vi "Dashboard Main.vi"() -> ()   [LabVIEW 2012]
uses:
  <vilib>/event_ctls.llb/eventvkey.ctl
  <vilib>/Utility/config.llb/Read Key (String).vi
  <vilib>/Utility/config.llb/Read Key (I32).vi
  <vilib>/Utility/config.llb/Write Key (String).vi
  <vilib>/Utility/config.llb/Write Key (I32).vi
  <vilib>/Utility/config.llb/NI_LVConfig.lvlib
panel:
  out "Battery Value":dbl(slide) scale=0.0..14.0 scale format="%#_2e"
  out "Battery":sgl(graph)
  in  "Camera Settings":T1={"Frate Rate"=30, "Compression"=30, "Size"=1} {"Frate Rate" scale=1.0..30.0; "Size" items=["640x480", "320x240", "160x120"]}
  out "Mode":T2(ring)=enum."Auto Disabled"
  out "Camera IP":string
  out "JS1 Z":dbl(slide) scale=-1.0..1.0 scale format="%#_2e"
  out "JS2 Z":dbl(slide) scale=-1.0..1.0 scale format="%#_2e"
  out "Joystick 1":cluster{"X":dbl, "Y":dbl}[](graph)
  out "Joystick 2":cluster{"X":dbl, "Y":dbl}[](graph)
  out "JS Buttons 1":T3
  out "JS Buttons 2":T3
  out "MotorSlide4":dbl(slide) scale=-1.0..1.0 scale format="%#_2e"
  out "MotorSlide3":dbl(slide) scale=-1.0..1.0 scale format="%#_2e"
  out "MotorSlide2":dbl(slide) scale=-1.0..1.0 scale format="%#_2e"
  in  "MotorName3":string="Front Left"
  in  "MotorName4":string="Front Right"
  in  "MotorName1":string="Rear Left"
  in  "MotorName2":string="Rear Right"
  out "MotorChart4":dbl(graph)
  out "MotorChart3":dbl(graph)
  out "MotorChart2":dbl(graph)
  out "MotorSlide1":dbl(slide) scale=-1.0..1.0 scale format="%#_2e"
  out "MotorChart1":dbl(graph)
  out "Robot IP":string
  in  "Dashboard Tab":T4(tab)
  in  "Checkbox 2":bool
  in  "Checkbox 1":bool
  in  "Slider 1":dbl(slide) scale=0.0..100.0
  in  "Target Choice":i8(knob) scale=0.0..2.0
  out "Numeric Target Info":dbl[](array[numeric])
  out "Image Out":T5(plugin-control)
  in  "Slider":dbl(slide) scale=0.0..100.0 scale format="%#_3g"
  in  "On/Off":bool caption="Solenoid"
  in  "Test Name":u16(ring) items=["Select the test to run...", "Example Test", "-------------------------------", "List of tests is built in robot code.", "Replace with your own automated tests."]
  in  "Test Tree":string(tree)
  in  "Motor":cluster{"Value":dbl, "Enable":bool} {"Value" scale=-1.0..1.0 scale format="%#_3g"}
  out "Progress":T6 {"Test Progress" scale=0.0..100.0}
  in  "Rev/Fwd":cluster{"Forward":bool, "Reverse":bool}
  in  "Ring":u16(ring) items=["Auto", "Fixed indoor", "Fixed outdoor 1", "Fixed outdoor 2", "Fixed fluorescent 1", "Fixed fluorescent 2", "Hold current"]
  in  "Listbox":i32(listbox)
  in  "Viewer":T7(tab)
  out "Mbps":dbl format="%#.1g"
  in  "Enable":bool
  in  "DB Camera Config":bool
  out "Mbps":bool
  out "fps":dbl format="%#.1g"
  out "Image Error Message":string="Timeout in Camera Communications"
  out "Camera Image":T5(plugin-control)
  out "Center Target":bool
  out "Buttons 1":cluster{"1":bool, "2":bool, "3":bool}
  out "Kinect 1":cluster{"X":dbl, "Y":dbl, "Z":dbl} {"X" scale=1.0..-1.0; "Y" scale=1.0..-1.0; "Z" scale=1.0..-1.0}
  out "Buttons 2":cluster{"1":bool, "2":bool, "3":bool}
  out "Kinect 2":cluster{"X":dbl, "Y":dbl, "Z":dbl} {"X" scale=1.0..-1.0; "Y" scale=1.0..-1.0; "Z" scale=1.0..-1.0}
  out "Version":string
  out "Skeleton Picture":picture
  out "Players":i8
  out "Tree":string(tree)
  # "Drive & Motors"
  # "Robot IP:"
  # "Customize by placing controls and indicators here and name to match\nDashboard Variables on robot."
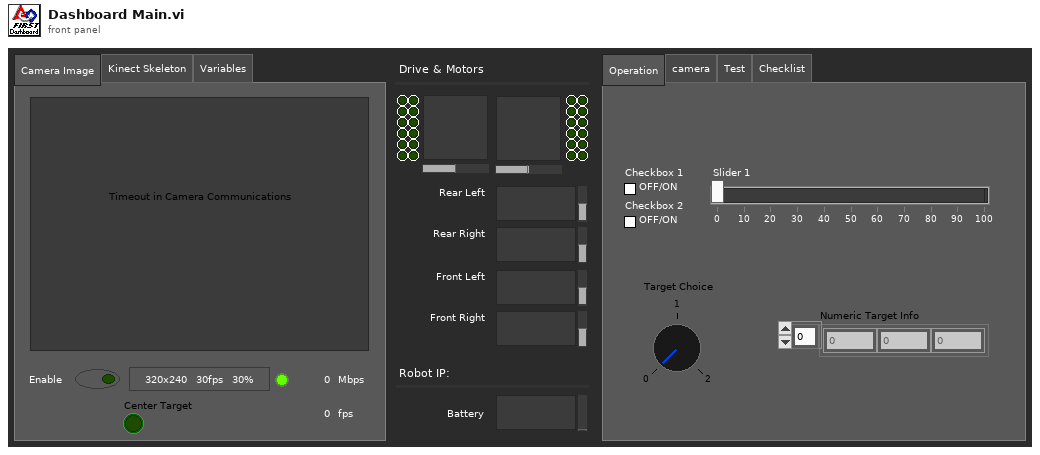
[diagram p1: front panel]
types:
  T1 = cluster{"Frate Rate":i32, "Compression":i32, "Size":u16}
  T2 = enum8{"Tele-Op Disabled", "Tele-Op Enabled", "Auto Disabled", "Auto Enabled", "Test Disabled", "Test Enabled", ""}
  T3 = cluster{bool, bool, bool, bool, bool, bool, bool, bool, bool, bool, bool, bool}
  T4 = enum32{"Operation", "camera", "Test", "Checklist"}
  T5 = typedef "IMAQ Image.ctl" = refnum<image>
  T6 = cluster{"Test Progress":u8, "Test Progress Text":string}
  T7 = enum32{"Camera Image", "Kinect Skeleton", "Variables"}
  T8 = typedef "Image Type" = u32
  T9 = typedef "LVBoundsTypeDef.ctl" = cluster{"Width":u32, "Height":u32}
  T10 = typedef "SkeletonTrackState.ctl" = enum32{"NotTracked", "PositionOnly", "Tracked"}
  T11 = cluster{"TrackingState":u8[], "Position":cluster{"x":sgl, "y":sgl, "z":sgl}, cluster{"x":sgl, "y":sgl, "z":sgl, sgl}[], "TrackState":T10}
  T12 = cluster{cluster{"ScaledToPercentRange":dbl, "ScaledToPercentRange":dbl, "ScaledToPercentRange":dbl}, cluster{bool, bool, bool}}[]
  T13 = cluster{cluster{"ScaledToPercentRange":dbl, "ScaledToPercentRange":dbl, "ScaledToPercentRange":dbl}, cluster{bool, bool, bool}}
  T14 = cluster{"ScaledToPercentRange":dbl, "ScaledToPercentRange":dbl, "ScaledToPercentRange":dbl}
  T15 = typedef "LVRectTypeDef.ctl" = cluster{"Left":i16, "Top":i16, "Right":i16, "Bottom":i16}
  T16 = cluster{"Competition mode":bool, "Robot Link":bool, "Autonomous":bool, "Enabled":bool, "E-Stop":bool, "Simulated":bool, "TestMode":bool, "Docked Window":bool}
  T17 = cluster{"Boolean Array[0]":bool, "Boolean Array[1]":bool, "Boolean Array[2]":bool, "Boolean Array[3]":bool, "Boolean Array[4]":bool, "Boolean Array[5]":bool, "Boolean Array[6]":bool, "Boolean Array[7]":bool, "Boolean Array[8]":bool, "Boolean Array[9]":bool, "Boolean Array[10]":bool, "Boolean Array[11]":bool}
  T18 = typedef "NI_LVConfig.lvlib/Config Data RefNum.ctl" = refnum<k1>
  T19 = typedef "eventvkey.ctl" = enum16{"ASCII", "Enter", "Return", "Shift", "Ctrl", "Alt", "Cmd", "Opt", "Caps", "NumLock", "Clear", "Break", "Up", "Down", "Left", "Right", "Insert", "Delete", "Home", "End", "PageUp", "PageDown", "Escape", "Help", "Pause", "ScrollLock", "F1", "F2", "F3", "F4", "F5", "F6", "F7", "F8", "F9", "F10", "F11", "F12", "F13", "F14", "F15", "F16", "F17", "F18", "F19", "F20", "F21", "F22", "F23", "F24", "Play", "VolumeUp", "VolumeDown", "Mute", "Two Byte Char"}
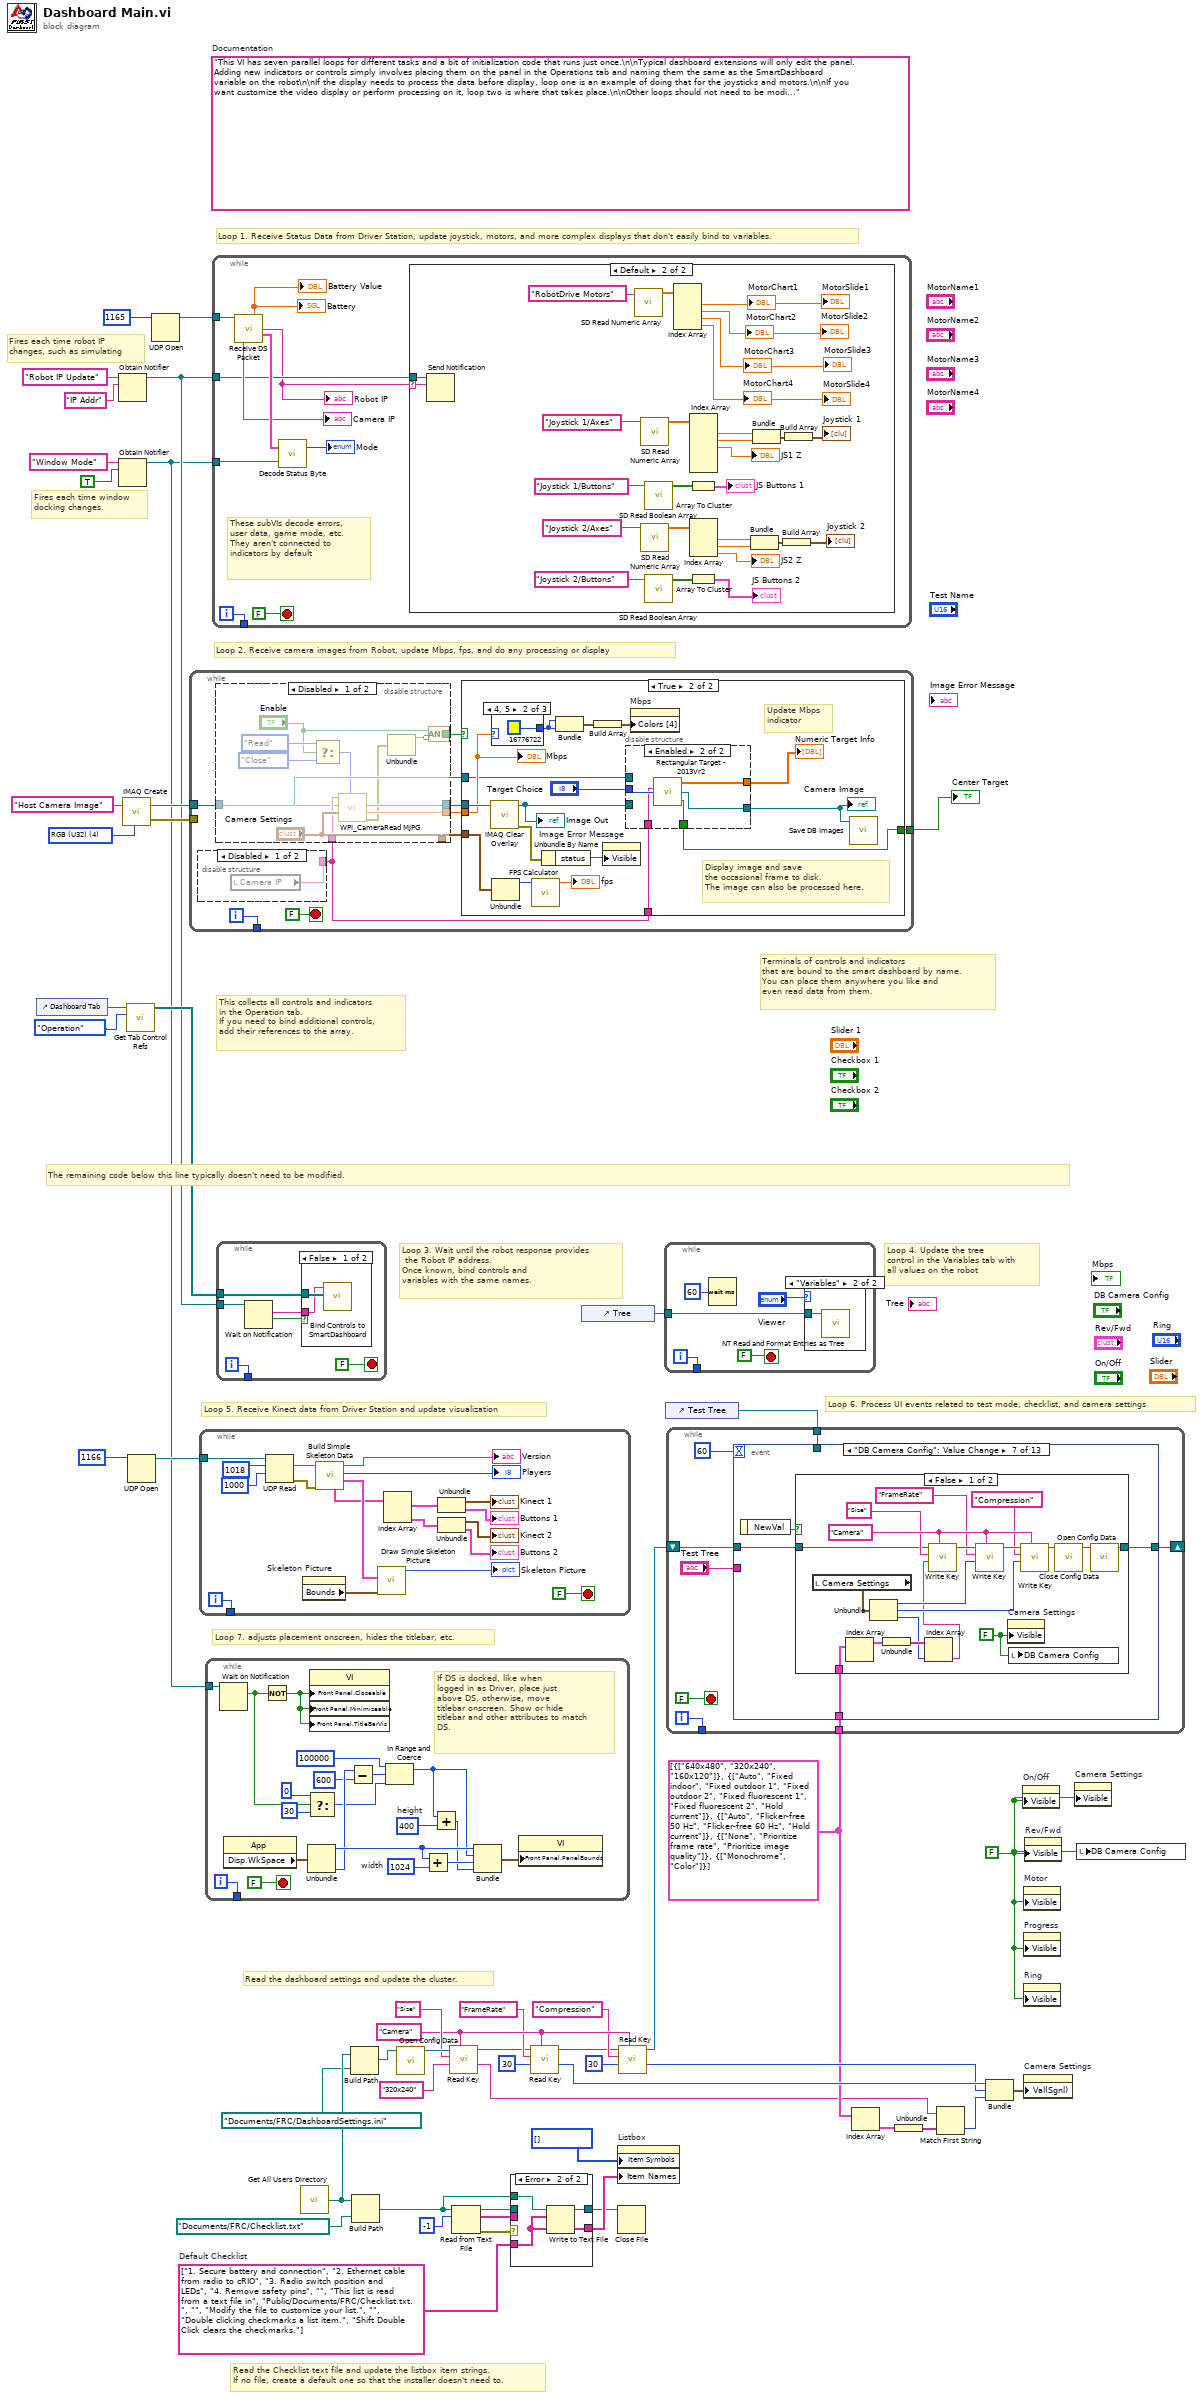
[diagram p0: block diagram]
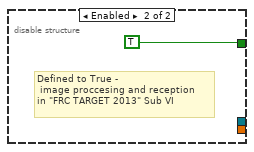
[diagram p3: hidden frame]
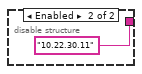
[diagram p4: hidden frame]
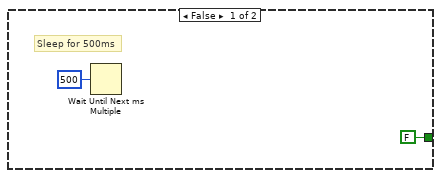
[diagram p5: hidden frame]
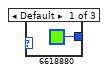
[diagram p7: hidden frame]
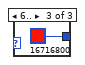
[diagram p8: hidden frame]
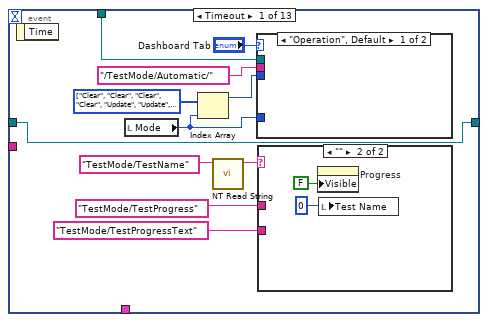
[diagram p10: hidden frame]
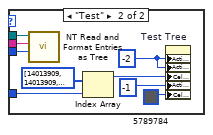
[diagram p11: hidden frame]
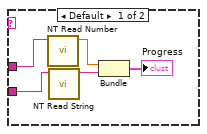
[diagram p12: hidden frame]
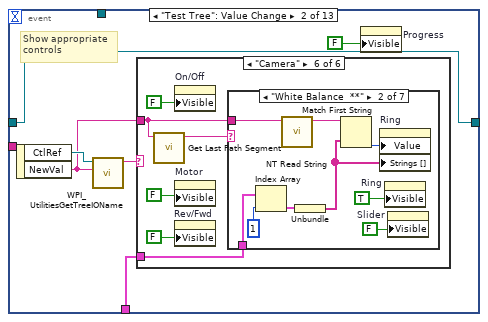
[diagram p13: hidden frame]
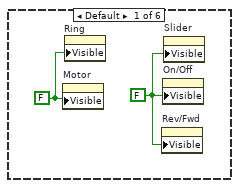
[diagram p14: hidden frame]
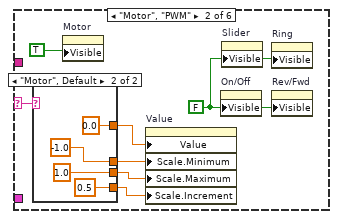
[diagram p15: hidden frame]
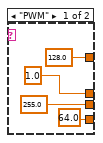
[diagram p16: hidden frame]
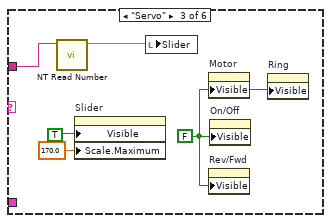
[diagram p17: hidden frame]
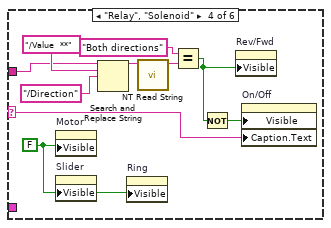
[diagram p18: hidden frame]
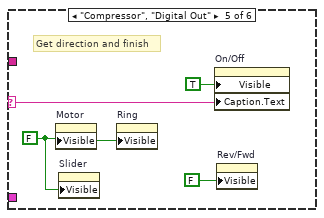
[diagram p19: hidden frame]
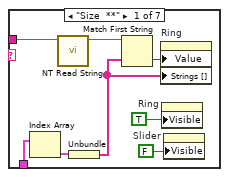
[diagram p20: hidden frame]
diagram:
  w22 = "Camera"
  w14 = cluster{string[]}[] [{["640x480", "320x240", "160x120"]}, {["Auto", "Fixed indoor", "Fixed outdoor 1", "Fixed outdoor 2", "Fixed fluorescent 1", "Fixed fluorescent 2", "Hold current"]}, {["Auto", "Flicker-free 50 Hz", "Flicker-free 60 Hz", "Hold current"]}, {["None", "Prioritize frame rate", "Prioritize image quality"]}, {["Monochrome", "Color"]}]
  w30 = string[] ["1. Secure battery and connection", "2. Ethernet cable from radio to cRIO", "3. Radio switch position and LEDs", "4. Remove safety pins", "", "This list is read from a text file in", "Public/Documents/FRC/Checklist.txt.", "", "Modify the file to customize your list.", "", "Double clicking checkmarks a list item.", "Shift Double Click clears the checkmarks."]  # Default Checklist
  w28 = FALSE ("Visible")
  (unwired) "This VI has seven parallel loops for different tasks and a bit of initialization code that runs just once.\n\nTypical dashboard extensions will only edit the panel. Adding new indicators or controls simply involves placing them on the panel in the Operations tab and naming them the same as the SmartDashboard variable on the robot\n\nIf the display needs to process the data before display, loop one is an example of doing that for the joysticks and motors.\n\nIf you want customize the video display or perform processing on it, loop two is where that takes place.\n\nOther loops should not need to be modified. They are pretty standard, and document the task they perform."  # Documentation
  w51 = T8 4 items=["Grayscale (U8)", "Grayscale (I16)", "Grayscale (SGL)", "Complex (CSG)", "RGB (U32)", "HSL (U32)", "RGB (U64)"] ("Image Type")
  # "Fires each time robot IP\nchanges, such as simulating"
  # "Fires each time window\ndocking changes."
  # "Read the Checklist text file and update the listbox item strings.\nIf no file, create a default one so that the installer doesn't need to."
  # "This collects all controls and indicators\nin the Operation tab.\nIf you need to bind additional controls,\nadd their references to the array."
  # "The remaining code below this line typically doesn't need to be modified."
  # "Loop 6. Process UI events related to test mode, checklist, and camera settings"
  # "Read the dashboard settings and update the cluster."
  # "Terminals of controls and indicators\nthat are bound to the smart dashboard by name.\nYou can place them anywhere you like and\neven read data from them."
  # "Loop 4. Update the tree\ncontrol in the Variables tab with\nall values on the robot"
  # "Loop 3. Wait until the robot response provides\n the Robot IP address.\nOnce known, bind controls and\nvariables with the same names."
  # "Loop 5. Receive Kinect data from Driver Station and update visualization"
  # "Loop 7. adjusts placement onscreen, hides the titlebar, etc."
  # "Loop 1. Receive Status Data from Driver Station, update joystick, motors, and more complex displays that don't easily bind to variables."
  # "Loop 2. Receive camera images from Robot, update Mbps, fps, and do any processing or display"
  n1 = control-ref of="Dashboard Tab"() -> (w44:refnum<vi>)
  n2 = Obtain Notifier(name (unnamed)="Robot IP Update", notification data type="IP Addr" ("name (unnamed)")) -> (notifier out=w41:refnum<notifier>)  [unwired: 2 in, 2 out]
  n3 = Obtain Notifier(name (unnamed)="Window Mode", notification data type=TRUE) -> (notifier out=w34:refnum<notifier>)  [unwired: 2 in, 2 out]
  n4 = call "IMAQ Create"("Image Name"="Host Camera Image", "Image Type"=w51) -> ("New Image"=w49:T5, "error out"=w48:errorcluster)  [unwired: 2 in, 1 out]
  n5 = call <vilib>:"Get Tab Control Refs.vi"("Page Index"=enum32{"Operation", "Test"}."Operation" ("Dashboard Tab"), "TabControl in"=w44) -> ("ControlsOnPage"=w45:refnum<vi>[])  [unwired: 9 in]
  n6 = UDP Open(11:u16 1166 ("port")) -> (port=w46:refnum<k16>)  [unwired: 2 in, 4 out]
  n7 = UDP Open(11:u16 1165 ("port")) -> (port=w52:refnum<k16>)  [unwired: 2 in, 4 out]
  n8 = while {
    tunnel: w49 -> [w56]
    tunnel: w48 -> [_]
    tunnel: [w61] -> _
    tunnel: [w54] -> w1
    i -> [w61]
    stop <- FALSE stop-if-true
    n9 = disable-structure shown="Disabled" {
      disable-tunnel: [w76 "10.22.30.11" ("camera IP")] -> w57
      frame Disabled {
        n10 = local read "Camera IP"() -> (w76:string)
      }
      frame Enabled {
      }
    }
    n11 = disable-structure shown="Disabled" {
      disable-tunnel: ["Camera Settings" _] -> w60
      disable-tunnel: [w73 _] -> w59
      disable-tunnel: [w72 _] -> w58
      disable-tunnel: [w65 TRUE] -> w55
      disable-tunnel: w57 -> [w64 _]
      disable-tunnel: w56 -> [w63 _]
      frame Disabled {
        n12 = Select(t=enum16{"Read", "Reopen", "Close"}."Read" ("Operation"), s="Enable", f=enum16{"Read", "Reopen", "Close"}."Close" ("Operation")) -> (s? t:f=w69:enum16{"Read", "Reopen", "Close"})
        n13 = call <vilib>:"WPI_CameraRead MJPG.vi"("Operation"=w69, "Camera Settings"="Camera Settings", "Image"=w63, "address"=w64) -> ("error out"=w68:errorcluster, "Bandwidth (kbps)"=w72:dbl, "Image Out"=w73:T5)  [unwired: 5 in]
        n14 = Unbundle(w68) -> ("status"=w66:bool)  [unwired: 2 out]
        n15 = Compound Arithmetic op=AND("Enable", invert w66) -> (w65:bool)
      }
      frame Enabled {
        # "Defined to True -\n image proccesing and reception \nin \"FRC TARGET 2013\" Sub VI"
      }
    }
    n16 = case shown="True" w55 {
      tunnel: w60 -> [_ w88]
      tunnel: w59 -> [_ w91]
      tunnel: w58 -> [_ w90]
      tunnel: w57 -> [_ w82]
      tunnel: w56 -> [_ w81]
      tunnel: [FALSE ("Center Target") w80] -> w54
      frame False {
        # "Sleep for 500ms"
        n17 = Wait Until Next ms Multiple(millisecond multiple=u32 500) -> ()  [unwired: 1 out]
      }
      frame True {
        # "Display image and save\nthe occasional frame to disk.\nThe image can also be processed here."
        # "Update Mbps\nindicator"
        n18 = call "IMAQ Clear Overlay"("Image"=w91) -> ("error out"=w95:errorcluster, "Image Out"=w85:T5)  [unwired: 2 in, 7 out]
        "Image Out" <- w85
        n19 = case shown="4, 5" w90 {
          tunnel: [u32 6618880 ("Color Box") u32 16776722 ("Color Box") u32 16716800 ("Color Box")] -> w92
          frame Default {
          }
          frame 4, 5 {
          }
          frame 6.. {
          }
        }
        n20 = Unbundle(w88) -> ("Frate Rate"=w87:i32)  [unwired: 2 out]
        n21 = call "FPS Calculator.vi"("Average Count"=w87) -> ("fps"=→"fps":dbl)  [unwired: 10 in]
        n22 = Unbundle By Name(w95) -> ("status"=w96:bool)
        n23 = Bundle("Color Box"=w92, "Color Box"=w92) -> (w94:cluster{"Color Box":u32, "Color Box":u32})  [unwired: 1 out]
        n24 = Build Array(w94) -> (w93:cluster{"Color Box":u32, "Color Box":u32}[])
        n25 = property on="Image Error Message" class="Str"("Visible"=w96) -> ()  [unwired: 2 in, 2 out]
        n26 = disable-structure shown="Enabled" {
          disable-tunnel: [w97 w102] -> w86
          disable-tunnel: w85 -> [w97 _]
          disable-tunnel: "Target Choice" -> [_ w101]
          disable-tunnel: [_ w100] -> w83
          disable-tunnel: w82 -> [_ w98]
          disable-tunnel: w81 -> [_ _]
          disable-tunnel: [_ w99] -> w80
          frame Disabled {
          }
          frame Enabled {
            n27 = call "Rectangular Target - 2013Vr2.vi"("Target Choice"=w101, "Camera IP Address"=w98) -> ("Center Target"=w99:bool, "Processed Image"=w102:T5, "Numeric Target Info"=w100:dbl[])  [unwired: 2 in]
          }
        }
        "Camera Image" <- w86
        "Numeric Target Info" <- w83
        n28 = property on="Mbps" class="Bool (strict)"("Colors [4]"=w93) -> ()  [unwired: 2 in, 2 out]
        n29 = call "Save DB Images.vi"("Image"=w86) -> ()  [unwired: 2 in, 1 out]
        "Mbps" <- w90
      }
    }
  }
  "Center Target" <- w1
  n30 = while {
    tunnel: w46 -> [w122]
    tunnel: [w107] -> _
    i -> [w107]
    stop <- FALSE stop-if-true
    n31 = UDP Read(connection ID=w122, max size (548)=1018 ("bytes to read"), timeout ms (25000)=1000) -> (data out=w116:string, error out=w106:errorcluster)  [unwired: 1 in, 3 out]
    n32 = property on="Skeleton Picture" class="Pict"() -> ("Bounds"=w118:T9)  [unwired: 2 in, 2 out]
    n33 = call "Build Simple Skeleton Data.vi"("error in (no error)"=w106, "data in"=w116) -> ("Skeleton Data"=w117:T11, "NumPlayers"=→"Players":i8, "Version String"=→"Version":string, "Simple Joystick Info"=w114:T12)  [unwired: 5 in, 1 out]
    n34 = call "Draw Simple Skeleton Picture.vi"("Bounds"=w118, "Simple Skeleton"=w117) -> ("new picture out"=→"Skeleton Picture":picture)  [unwired: 9 in]
    n35 = Index Array(array=w114) -> (element #1=w113:T13, element #2=w112:T13)  [unwired: 2 in]
    n36 = Unbundle(w113) -> (→"Kinect 1":T14, →"Buttons 1":cluster{bool, bool, bool})
    n37 = Unbundle(w112) -> (→"Kinect 2":T14, →"Buttons 2":cluster{bool, bool, bool})
  }
  n38 = while {
    tunnel: w34 -> [w143]
    tunnel: [w141] -> _
    i -> [w141]
    stop <- FALSE stop-if-true
    w133 = 1024  # width
    w136 = 400  # height
    # "If DS is docked, like when\nlogged in as Driver, place just\nabove DS, otherwise, move\ntitlebar onscreen. Show or hide\ntitlebar and other attributes to match\nDS."
    n39 = Wait on Notification(notifier=w143) -> (notification=w128:bool)  [unwired: 3 in, 3 out]
    n40 = property class="App"() -> ("Disp.WkSpace"=w139:T15)  [unwired: 2 in, 2 out]
    n41 = Not(x=w128) -> (.not. x?=w142:bool)
    n42 = Unbundle(w139) -> ("Left"=w137:i16, "Bottom"=w134:i16)  [unwired: 2 out]
    n43 = Select(t=0, s=w128, f=30) -> (s? t:f=w127:i32)
    n44 = property class="VI"("Front Panel.Closeable"=w142, "Front Panel.Minimizeable"=w142, "Front Panel.TitleBarVis"=w142) -> ()  [unwired: 2 in, 2 out]
    n45 = Subtract(x=w134, y=600) -> (x-y=w131:i32)
    n46 = In Range and Coerce(upper limit=100000, x=w131, lower limit=w127) -> (coerced(x)=w125:i32)  [unwired: 1 out]
    n47 = Add(x=w137, y=w133) -> (x+y=w138:i32)
    n48 = Add(x=w125, y=w136) -> (x+y=w135:i32)
    n49 = Bundle("Left"=w137, w125, w138, w135) -> (w140:cluster{"Left":i16, i32, i32, i32})  [unwired: 1 out]
    n50 = property class="VI"("Front Panel.PanelBounds"=w140) -> ()  [unwired: 2 in, 2 out]
  }
  n51 = while {
    tunnel: w52 -> [w152]
    tunnel: w41 -> [w146]
    tunnel: w34 -> [w150]
    tunnel: [w147] -> _
    i -> [w147]
    stop <- FALSE stop-if-true
    # "These subVIs decode errors, user data, game mode, etc.\nThey aren't connected to indicators by default"
    n52 = call "Receive DS Packet.vi"("Recv Socket"=w152) -> ("Battery"=→"Battery" →"Battery Value":sgl, "Robot IP Address"=w145:string, "Status"=w153:T16, "Camera IP Address"=→"Camera IP":string)  [unwired: 1 in, 10 out]
    "Robot IP" <- w145
    n53 = call "Decode Status Byte.vi"("Window Mode Notifier"=w150, "Status"=w153) -> ("Mode"=→"Mode":T2)  [unwired: 1 out]
    n54 = case shown="Default" w145 {
      selector: w145 -> [_ w155]
      tunnel: w146 -> [_ w156]
      frame "0.0.0.0" {
        # "Robot not responding, don't poll the variables"
      }
      frame Default {
        n55 = Send Notification(notification=w155, notifier=w156) -> ()  [unwired: 1 in, 2 out]
        n56 = call <vilib>:"SD Read Numeric Array.vi"("Name"="RobotDrive Motors") -> ("Numeric Array"=w179:dbl[])  [unwired: 8 in, 2 out]
        n57 = call <vilib>:"SD Read Numeric Array.vi"("Name"="Joystick 1/Axes") -> ("Numeric Array"=w172:dbl[])  [unwired: 8 in, 2 out]
        n58 = call <vilib>:"SD Read Numeric Array.vi"("Name"="Joystick 2/Axes") -> ("Numeric Array"=w166:dbl[])  [unwired: 8 in, 2 out]
        n59 = call <vilib>:"SD Read Boolean Array.vi"("Name"="Joystick 1/Buttons") -> ("Boolean Array"=w174:bool[])  [unwired: 8 in, 2 out]
        n60 = call <vilib>:"SD Read Boolean Array.vi"("Name"="Joystick 2/Buttons") -> ("Boolean Array"=w165:bool[])  [unwired: 8 in, 2 out]
        n61 = Index Array(array=w179) -> (element #1=→"MotorChart1" →"MotorSlide1":dbl, element #2=→"MotorSlide2" →"MotorChart2":dbl, element #3=→"MotorChart3" →"MotorSlide3":dbl, element #4=→"MotorChart4" →"MotorSlide4":dbl)  [unwired: 4 in]
        n62 = Array To Cluster(array=w174) -> (cluster=→"JS Buttons 1":T17)
        n63 = Array To Cluster(array=w165) -> (cluster=→"JS Buttons 2":T17)
        n64 = Index Array(array=w172) -> (element #1=w169:dbl, element #2=w170:dbl, element #3=→"JS1 Z":dbl)  [unwired: 6 in, 3 out]
        n65 = Index Array(array=w166) -> (element #1=w161:dbl, element #2=w160:dbl, element #3=→"JS2 Z":dbl)  [unwired: 3 in]
        n66 = Bundle("Numeric"=w161, "Numeric"=w160) -> (w162:cluster{"Numeric":dbl, "Numeric":dbl})  [unwired: 1 in]
        n67 = Bundle("Numeric"=w169, "Numeric"=w170) -> (w168:cluster{"Numeric":dbl, "Numeric":dbl})  [unwired: 1 in]
        n68 = Build Array(w162) -> (→"Joystick 2":cluster{"Numeric":dbl, "Numeric":dbl}[])
        n69 = Build Array(w168) -> (→"Joystick 1":cluster{"Numeric":dbl, "Numeric":dbl}[])
      }
    }
  }
  n70 = while {
    tunnel: w45 -> [w188]
    tunnel: w41 -> [w185]
    tunnel: [w183] -> _
    i -> [w183]
    stop <- FALSE stop-if-true
    n71 = Wait on Notification(notifier=w185) -> (notification=w184:string, timed out?=w186:bool)  [unwired: 3 in, 2 out]
    n72 = case shown="False" w186 {
      tunnel: w188 -> [w190 _]
      tunnel: w184 -> [w189 _]
      frame False {
        n73 = call <vilib>:"Bind Controls to SmartDashboard.vi"("Bound Control Refs"=w190, "Server IP Address"=w189) -> ()  [unwired: 10 in]
      }
      frame True {
      }
    }
  }
  n74 = call "Get All Users Directory.vi"() -> ("All User Path"=w27:path)
  n75 = Build Path(base path=w27, name or relative path=path "Documents/FRC/DashboardSettings.ini") -> (appended path=w26:path)
  n76 = Build Path(base path=w27, name or relative path=path "Documents/FRC/Checklist.txt") -> (appended path=w31:path)
  n77 = call <vilib>:"Open Config Data.vi"("configuration file path"=w26) -> ("refnum"=w25:T18)  [unwired: 8 in, 2 out]
  n78 = call-poly <vilib>:"Read Key.vi"("section"=w22, "default value"="320x240", "key"="Size", "refnum"=w25) -> ("value"=w12:string, "refnum out"=w7:T18)  [unwired: 2 in, 4 out]
  n79 = Read from Text File(file (use dialog)=w31, count=-1 ("timeout ms (25000)")) -> (refnum out=w9:refnum<file>, text=w32:string[], error out=w33:errorcluster)  [unwired: 2 in, 1 out]
  n80 = case shown="Error" w33 {
    tunnel: w32 -> [w192 _]
    tunnel: [w192 w194] -> w29
    tunnel: w30 -> [_ w194]
    tunnel: w31 -> [_ w195]
    tunnel: [w191 w193] -> w8
    tunnel: w9 -> [w191 _]
    frame No Error {
    }
    frame Error {
      n81 = Write to Text File(file (use dialog)=w195, text=w194) -> (refnum out=w193:refnum<file>)  [unwired: 2 in, 2 out]
    }
  }
  n82 = call-poly <vilib>:"Read Key.vi"("section"=w22, "default value"=30, "key"="FrameRate", "refnum"=w7) -> ("value"=w17:i32, "refnum out"=w6:T18)  [unwired: 1 in, 5 out]
  n83 = control-ref of="Tree"() -> (w3:refnum<vi>)
  n84 = property on="Listbox" class="LstBox (strict)"("Item Symbols"=i32[] [], "Item Names"=w29) -> ()  [unwired: 2 in, 2 out]
  n85 = Close File(refnum=w8) -> ()  [unwired: 1 in, 2 out]
  n86 = call-poly <vilib>:"Read Key.vi"("section"=w22, "default value"=30, "key"="Compression", "refnum"=w6) -> ("value"=w16:i32, "refnum out"=w4:T18)  [unwired: 1 in, 5 out]
  n87 = while {
    tunnel: [w197] -> _
    tunnel: w3 -> [w196]
    i -> [w197]
    stop <- FALSE stop-if-true
    n88 = Wait (ms)(milliseconds to wait=u32 60) -> ()  [unwired: 1 out]
    n89 = case shown="\"Variables\"" "Viewer" {
      tunnel: w196 -> [_ w201]
      frame Default {
      }
      frame "Variables" {
        n90 = call <vilib>:"NT Read and Format Entries as Tree.vi"("Tree Refnum"=w201) -> ()  [unwired: 9 in, 2 out]
      }
    }
  }
  n91 = control-ref of="Test Tree"() -> (w2:refnum<vi>)
  n92 = while {
    tunnel: w14 -> [w206]
    shift-right: [w205] -> _
    shift-left: w4 -> [w204]
    tunnel: [w203] -> _
    tunnel: w2 -> [w202]
    i -> [w203]
    stop <- FALSE stop-if-true
    n93 = event shown="[6] \"DB Camera Config\": Value Change" {
      selector: _ -> [_ _ _ _ _ _ _ _ _ _ _ _ _]
      dyn-events: _ -> [_ _ _ _ _ _ _ _ _ _ _ _ _]
      timeout: u32 60 ("milliseconds to wait") -> [_ _ _ _ _ _ _ _ _ _ _ _ _]
      tunnel: w202 -> [w216 _ _ _ _ _ _ _ _ _ _ _ _]
      tunnel: "Test Tree" -> [_ _ _ _ _ _ _ _ w410 w418 w420 w424 w432]
      tunnel: w206 -> [_ w238 _ _ _ _ w374 w404 _ _ _ _ _]
      tunnel: [w210 w237 _ w340 w348 w360 w373 w397 w409 w416 w419 w423 w431] -> w205
      tunnel: w204 -> [w210 w237 _ w340 w348 w360 w372 w397 w409 w416 w419 w423 w431]
      event Timeout {
        w215 = enum16{"Update", "Clear"}[] [enum."Clear", enum."Clear", enum."Clear", enum."Clear", enum."Update", enum."Update", enum."Clear"] items=["Update", "Clear"]
        n94 = event-data() -> ()  [unwired: 1 in, 1 out]
        n95 = local read "Mode"() -> (w213:T2)
        n96 = Index Array(array=w215, index=w213) -> (element=w214:enum16{"Update", "Clear"})
        n97 = call <vilib>:"NT Read String.vi"("Name"="TestMode/TestName") -> ("String"=w219:string)  [unwired: 9 in, 1 out]
        n98 = case shown="\"Operation\", Default" "Dashboard Tab" {
          tunnel: w216 -> [_ w229]
          tunnel: "/TestMode/Automatic/" ("Name Pattern") -> [_ w228]
          tunnel: w214 -> [_ w227]
          tunnel: w213 -> [_ w225]
          frame "Operation", Default {
          }
          frame "Test" {
            w224 = -2 ("Active Item:Row Number")
            n99 = call <vilib>:"NT Read and Format Entries as Tree.vi"("Operation"=w227, "Name Pattern"=w228, "Tree Refnum"=w229) -> ()  [unwired: 7 in, 2 out]
            n100 = Index Array(array=u32[] [14013909, 14013909, 14013909, 14013909, 14013909, 16777215, 14013909], index=w225) -> (element=w223:u32)
            n101 = property on="Test Tree" class="Tree (strict)"("Active Item Row Number"=w224, "ActiveColNum"=w224, "CellBG"=w223, "Active Item Row Number"=-1 ("Active Item:Row Number"), "CellBG"=u32 5789784 ("Color Box")) -> ()  [unwired: 2 in, 2 out]
          }
        }
        n102 = case shown="\"\"" w219 {
          tunnel: "TestMode/TestProgress" ("Name") -> [w231 _]
          tunnel: "TestMode/TestProgressText" ("Name") -> [w230 _]
          frame Default {
            n103 = call <vilib>:"NT Read Number.vi"("Name"=w231) -> ("Numeric"=w232:dbl)  [unwired: 9 in, 1 out]
            n104 = call <vilib>:"NT Read String.vi"("Name"=w230) -> ("String"=w233:string)  [unwired: 9 in, 1 out]
            n105 = Bundle("Numeric"=w232, "String"=w233) -> (→"Progress":cluster{"Numeric":dbl, "String":string})  [unwired: 1 in]
          }
          frame "" {
            n106 = property on="Progress" class="Clust (strict)"("Visible"=FALSE) -> ()  [unwired: 2 in, 2 out]
            n107 = local write "Test Name"(u16 0) -> ()
          }
        }
      }
      event "Test Tree": Value Change {
        # "Show appropriate\ncontrols"
        n108 = event-data() -> ("CtlRef"=w241:refnum<vi>, "NewVal"=w239:string)  [unwired: 1 in]
        n109 = call <vilib>:"WPI_UtilitiesGetTreeIOName.vi"("NewVal"=w239, "TreeControl in"=w241) -> ("I/O Name"=w242:string)  [unwired: 9 in]
        n110 = case shown="\"Camera\"" w242 {
          selector: w242 -> [_ w249 _ w267 w276 _]
          tunnel: w239 -> [_ _ w264 w266 _ w283]
          tunnel: w238 -> [_ _ _ _ _ w282]
          frame Default {
            w244 = FALSE ("Visible")
            w243 = FALSE ("Visible")
            n111 = property on="Motor" class="Clust (strict)"("Visible"=w243) -> ()  [unwired: 2 in, 2 out]
            n112 = property on="Ring" class="Ring (strict)"("Visible"=w243) -> ()  [unwired: 2 in, 2 out]
            n113 = property on="Rev/Fwd" class="Clust (strict)"("Visible"=w244) -> ()  [unwired: 2 in, 2 out]
            n114 = property on="On/Off" class="Bool (strict)"("Visible"=w244) -> ()  [unwired: 2 in, 2 out]
            n115 = property on="Slider" class="Slide (strict)"("Visible"=w244) -> ()  [unwired: 2 in, 2 out]
          }
          frame "Motor", "PWM" {
            w250 = FALSE ("Visible")
            n116 = case shown="\"Motor\", Default" w249 {
              tunnel: [1.0 ("Value") -1.0 ("Value")] -> w248
              tunnel: [255.0 ("Value") 1.0 ("Value")] -> w247
              tunnel: [128.0 ("Value") 0.0 ("Value")] -> w246
              tunnel: [64.0 ("Value") 0.5 ("Value")] -> w245
              frame "PWM" {
              }
              frame "Motor", Default {
              }
            }
            n117 = property on="Motor" class="Clust (strict)"("Visible"=TRUE) -> ()  [unwired: 2 in, 2 out]
            n118 = property on="Value" class="Slide (strict)"("Value"=w246, "Scale.Minimum"=w248, "Scale.Maximum"=w247, "Scale.Increment"=w245) -> ()  [unwired: 2 in, 2 out]
            n119 = property on="On/Off" class="Bool (strict)"("Visible"=w250) -> ()  [unwired: 2 in, 2 out]
            n120 = property on="Slider" class="Slide (strict)"("Visible"=w250) -> ()  [unwired: 2 in, 2 out]
            n121 = property on="Ring" class="Ring (strict)"("Visible"=w250) -> ()  [unwired: 2 in, 2 out]
            n122 = property on="Rev/Fwd" class="Clust (strict)"("Visible"=w250) -> ()  [unwired: 2 in, 2 out]
          }
          frame "Servo" {
            w262 = FALSE ("Visible")
            n123 = call <vilib>:"NT Read Number.vi"("Name"=w264) -> ("Numeric"=w263:dbl)  [unwired: 9 in, 1 out]
            n124 = property on="Slider" class="Slide (strict)"("Visible"=TRUE, "Scale.Maximum"=170.0 ("Scale.Range:Maximum")) -> ()  [unwired: 2 in, 2 out]
            n125 = local write "Slider"(w263) -> ()
            n126 = property on="Motor" class="Clust (strict)"("Visible"=w262) -> ()  [unwired: 2 in, 2 out]
            n127 = property on="Rev/Fwd" class="Clust (strict)"("Visible"=w262) -> ()  [unwired: 2 in, 2 out]
            n128 = property on="On/Off" class="Bool (strict)"("Visible"=w262) -> ()  [unwired: 2 in, 2 out]
            n129 = property on="Ring" class="Ring (strict)"("Visible"=w262) -> ()  [unwired: 2 in, 2 out]
          }
          frame "Relay", "Solenoid" {
            w265 = FALSE ("Visible")
            n130 = property on="Motor" class="Clust (strict)"("Visible"=w265) -> ()  [unwired: 2 in, 2 out]
            n131 = property on="Slider" class="Slide (strict)"("Visible"=w265) -> ()  [unwired: 2 in, 2 out]
            n132 = Search and Replace String(input string=w266, search string="/Value  **", replace string="/Direction") -> (result string=w272:string)  [unwired: 5 in, 3 out]
            n133 = property on="Ring" class="Ring (strict)"("Visible"=w265) -> ()  [unwired: 2 in, 2 out]
            n134 = call <vilib>:"NT Read String.vi"("Name"=w272) -> ("String"=w270:string)  [unwired: 9 in, 1 out]
            n135 = Equal?(x="Both directions", y=w270) -> (x = y?=w268:bool)
            n136 = Not(x=w268) -> (.not. x?=w269:bool)
            n137 = property on="Rev/Fwd" class="Clust (strict)"("Visible"=w268) -> ()  [unwired: 2 in, 2 out]
            n138 = property on="On/Off" class="Bool (strict)"("Visible"=w269, "Caption.Text"=w267) -> ()  [unwired: 2 in, 2 out]
          }
          frame "Compressor", "Digital Out" {
            w275 = FALSE ("Visible")
            # "Get direction and finish"
            n139 = property on="Motor" class="Clust (strict)"("Visible"=w275) -> ()  [unwired: 2 in, 2 out]
            n140 = property on="Slider" class="Slide (strict)"("Visible"=w275) -> ()  [unwired: 2 in, 2 out]
            n141 = property on="Ring" class="Ring (strict)"("Visible"=w275) -> ()  [unwired: 2 in, 2 out]
            n142 = property on="On/Off" class="Bool (strict)"("Visible"=TRUE, "Caption.Text"=w276) -> ()  [unwired: 2 in, 2 out]
            n143 = property on="Rev/Fwd" class="Clust (strict)"("Visible"=FALSE) -> ()  [unwired: 2 in, 2 out]
          }
          frame "Camera" {
            n144 = call <vilib>:"Get Last Path Segment.vi"("String in"=w283) -> ("String out"=w284:string)  [unwired: 10 in]
            n145 = property on="On/Off" class="Bool (strict)"("Visible"=FALSE) -> ()  [unwired: 2 in, 2 out]
            n146 = property on="Motor" class="Clust (strict)"("Visible"=FALSE) -> ()  [unwired: 2 in, 2 out]
            n147 = property on="Rev/Fwd" class="Clust (strict)"("Visible"=FALSE) -> ()  [unwired: 2 in, 2 out]
            n148 = case shown="\"White Balance  **\"" w284 {
              tunnel: w283 -> [w290 w299 w308 w317 w326 _ w332]
              tunnel: w282 -> [w288 w296 w305 w314 w323 _ _]
              frame "Size  **" {
                n149 = Index Array(array=w288) -> (element=w287:cluster{string[]})  [unwired: 1 in]
                n150 = call <vilib>:"NT Read String.vi"("Name"=w290) -> ("String"=w289:string)  [unwired: 9 in, 1 out]
                n151 = Unbundle(w287) -> (w285:string[])
                n152 = Match First String(2:w285, 3:w289) -> (0:w286:i32)  [unwired: 1 out]
                n153 = property on="Ring" class="Ring (strict)"("Value"=w286, "Strings []"=w285) -> ()  [unwired: 2 in, 2 out]
                n154 = property on="Ring" class="Ring (strict)"("Visible"=TRUE) -> ()  [unwired: 2 in, 2 out]
                n155 = property on="Slider" class="Slide (strict)"("Visible"=FALSE) -> ()  [unwired: 2 in, 2 out]
              }
              frame "White Balance  **" {
                n156 = Index Array(array=w296, index=1) -> (element=w297:cluster{string[]})
                n157 = call <vilib>:"NT Read String.vi"("Name"=w299) -> ("String"=w298:string)  [unwired: 9 in, 1 out]
                n158 = Unbundle(w297) -> (w294:string[])
                n159 = Match First String(2:w294, 3:w298) -> (0:w293:i32)  [unwired: 1 out]
                n160 = property on="Ring" class="Ring (strict)"("Value"=w293, "Strings []"=w294) -> ()  [unwired: 2 in, 2 out]
                n161 = property on="Ring" class="Ring (strict)"("Visible"=TRUE) -> ()  [unwired: 2 in, 2 out]
                n162 = property on="Slider" class="Slide (strict)"("Visible"=FALSE) -> ()  [unwired: 2 in, 2 out]
              }
              frame "Exposure  **" {
                n163 = Index Array(array=w305, index=2) -> (element=w306:cluster{string[]})
                n164 = call <vilib>:"NT Read String.vi"("Name"=w308) -> ("String"=w307:string)  [unwired: 9 in, 1 out]
                n165 = Unbundle(w306) -> (w302:string[])
                n166 = Match First String(2:w302, 3:w307) -> (0:w303:i32)  [unwired: 1 out]
                n167 = property on="Ring" class="Ring (strict)"("Value"=w303, "Strings []"=w302) -> ()  [unwired: 2 in, 2 out]
                n168 = property on="Ring" class="Ring (strict)"("Visible"=TRUE) -> ()  [unwired: 2 in, 2 out]
                n169 = property on="Slider" class="Slide (strict)"("Visible"=FALSE) -> ()  [unwired: 2 in, 2 out]
              }
              frame "Exposure Priority  **" {
                n170 = Index Array(array=w314, index=3) -> (element=w315:cluster{string[]})
                n171 = call <vilib>:"NT Read String.vi"("Name"=w317) -> ("String"=w316:string)  [unwired: 9 in, 1 out]
                n172 = Unbundle(w315) -> (w311:string[])
                n173 = Match First String(2:w311, 3:w316) -> (0:w312:i32)  [unwired: 1 out]
                n174 = property on="Ring" class="Ring (strict)"("Value"=w312, "Strings []"=w311) -> ()  [unwired: 2 in, 2 out]
                n175 = property on="Ring" class="Ring (strict)"("Visible"=TRUE) -> ()  [unwired: 2 in, 2 out]
                n176 = property on="Slider" class="Slide (strict)"("Visible"=FALSE) -> ()  [unwired: 2 in, 2 out]
              }
              frame "Color Enable  **" {
                n177 = Index Array(array=w323, index=4) -> (element=w324:cluster{string[]})
                n178 = call <vilib>:"NT Read String.vi"("Name"=w326) -> ("String"=w325:string)  [unwired: 9 in, 1 out]
                n179 = Unbundle(w324) -> (w320:string[])
                n180 = Match First String(2:w320, 3:w325) -> (0:w321:i32)  [unwired: 1 out]
                n181 = property on="Ring" class="Ring (strict)"("Value"=w321, "Strings []"=w320) -> ()  [unwired: 2 in, 2 out]
                n182 = property on="Ring" class="Ring (strict)"("Visible"=TRUE) -> ()  [unwired: 2 in, 2 out]
                n183 = property on="Slider" class="Slide (strict)"("Visible"=FALSE) -> ()  [unwired: 2 in, 2 out]
              }
              frame Default {
                n184 = property on="Ring" class="Ring (strict)"("Visible"=FALSE) -> ()  [unwired: 2 in, 2 out]
                n185 = property on="Slider" class="Slide (strict)"("Visible"=FALSE) -> ()  [unwired: 2 in, 2 out]
              }
              frame "Brightness  **", "Color Level  **", "Compression  **", "FPS  **", "Sharpness  **" {
                n186 = call <vilib>:"NT Read Number.vi"("Name"=w332) -> ("Numeric"=w331:dbl)  [unwired: 9 in, 1 out]
                n187 = local write "Slider"(w331) -> ()
                n188 = property on="Slider" class="Slide (strict)"("Visible"=TRUE, "Scale.Maximum"=100.0 ("Scale.Range:Maximum")) -> ()  [unwired: 2 in, 2 out]
                n189 = property on="Ring" class="Ring (strict)"("Visible"=FALSE) -> ()  [unwired: 2 in, 2 out]
              }
            }
          }
        }
        n190 = property on="Progress" class="Clust (strict)"("Visible"=FALSE) -> ()  [unwired: 2 in, 2 out]
      }
      event "Test Name": Mouse Enter {
        # "Populate the ring with the list of tests"
        n191 = event-data() -> ()  [unwired: 1 in, 1 out]
        n192 = call <vilib>:"NT Read String Array.vi"("Name"="TestMode/TestList") -> ("String Array"=w339:string[])  [unwired: 9 in, 1 out]
        n193 = Build Array (concatenate)("Select the test to run...", w339) -> (w338:string[])
        n194 = property on="Test Name" class="Ring (strict)"("Strings []"=w338) -> ()  [unwired: 2 in, 2 out]
      }
      event "Test Name": Value Change {
        w341 = FALSE ("Visible")
        # "Tell the robot the test name to run"
        n195 = event-data() -> ("NewVal"=w345:u16)  [unwired: 1 in]
        n196 = property on="Test Name" class="Ring (strict)"() -> ("Strings []"=w346:string[])  [unwired: 2 in, 2 out]
        n197 = local write "Progress"(T6 {"Test Progress"=0, "Test Progress Text"=""} ("Progress")) -> ()
        n198 = Index Array(array=w346, index=w345) -> (element=w344:string)
        n199 = call <vilib>:"NT Write String.vi"("String"=w344, "Name"="TestMode/TestName") -> ()  [unwired: 9 in, 1 out]
        n200 = property on="Progress" class="Clust (strict)"("Visible"=TRUE) -> ()  [unwired: 2 in, 2 out]
        n201 = property on="Motor" class="Clust (strict)"("Visible"=w341) -> ()  [unwired: 2 in, 2 out]
        n202 = property on="Slider" class="Slide (strict)"("Visible"=w341) -> ()  [unwired: 2 in, 2 out]
        n203 = property on="On/Off" class="Bool (strict)"("Visible"=w341) -> ()  [unwired: 2 in, 2 out]
        n204 = property on="Rev/Fwd" class="Clust (strict)"("Visible"=w341) -> ()  [unwired: 2 in, 2 out]
        n205 = property on="Ring" class="Ring (strict)"("Visible"=w341) -> ()  [unwired: 2 in, 2 out]
      }
      event "Listbox": Double Click {
        n206 = event-data() -> ("PlatMods.Shift"=w349:bool, "Row"=w351:i32)  [unwired: 1 in]
        n207 = case shown="False" w349 {
          tunnel: w351 -> [w355 _]
          tunnel: 1 -> [w354 _]
          frame False {
            n208 = property on="Listbox" class="LstBox (strict)"() -> ("Item Symbols"=w353:i32[])  [unwired: 2 in, 2 out]
            n209 = Replace Array Subset(array=w353, new element=w354, index=w355) -> (w352:i32[])
            n210 = property on="Listbox" class="LstBox (strict)"("Item Symbols"=w352) -> ()  [unwired: 2 in, 2 out]
          }
          frame True {
            w356 = 0 ("Top Row")
            n211 = property on="Listbox" class="LstBox (strict)"() -> ("Number of Rows"=w358:u32)  [unwired: 2 in, 2 out]
            n212 = Initialize Array(0, w358) -> (w357:i32[])
            n213 = property on="Listbox" class="LstBox (strict)"("Top Row"=w356, "Value"=w356, "Item Symbols"=w357) -> ()  [unwired: 2 in, 2 out]
          }
        }
      }
      event "Listbox": Key Down {
        n214 = event-data() -> ("VKey"=w362:T19)  [unwired: 1 in]
        n215 = case shown="\"Left\", \"Right\"" w362 {
          selector: w362 -> [w367 _]
          tunnel: eventvkey."Left" ("VKey") -> [w365 _]
          frame "Left", "Right" {
            n216 = Equal?(x=w365, y=w367) -> (x = y?=w366:bool)
            n217 = Select(t=0, s=w366, f=1) -> (s? t:f=w368:i32)
            n218 = property on="Listbox" class="LstBox (strict)"() -> ("Item Symbols"=w371:i32[])  [unwired: 2 in, 2 out]
            n219 = Replace Array Subset(array=w371, new element=w368, index="Listbox") -> (w370:i32[])
            n220 = property on="Listbox" class="LstBox (strict)"("Item Symbols"=w370) -> ()  [unwired: 2 in, 2 out]
          }
          frame Default {
          }
        }
      }
      event "DB Camera Config": Value Change {
        n221 = event-data() -> ("NewVal"=w375:bool)  [unwired: 1 in]
        n222 = case shown="False" w375 {
          tunnel: w374 -> [w384 _]
          tunnel: [w377 w395] -> w373
          tunnel: w372 -> [w376 w395]
          frame False {
            w391 = "Camera"
            w394 = FALSE ("Visible")
            n223 = local read "Camera Settings"() -> (w383:T1)
            n224 = Index Array(array=w384) -> (element=w387:cluster{string[]})  [unwired: 1 in]
            n225 = Unbundle(w383) -> ("Frate Rate"=w382:i32, "Compression"=w381:i32, "Size"=w385:u16)
            n226 = Unbundle(w387) -> (w386:string[])
            n227 = Index Array(array=w386, index=w385) -> (element=w380:string)
            n228 = call-poly <vilib>:"Write Key.vi"("section"=w391, "value"=w380, "key"="Size", "refnum"=w376) -> ("refnum out"=w393:T18)  [unwired: 2 in, 5 out]
            n229 = call-poly <vilib>:"Write Key.vi"("section"=w391, "value"=w382, "key"="FrameRate", "refnum"=w393) -> ("refnum out"=w392:T18)  [unwired: 1 in, 6 out]
            n230 = property on="Camera Settings" class="Clust (strict)"("Visible"=w394) -> ()  [unwired: 2 in, 2 out]
            n231 = local write "DB Camera Config"(w394) -> ()
            n232 = call-poly <vilib>:"Write Key.vi"("section"=w391, "value"=w381, "key"="Compression", "refnum"=w392) -> ("refnum out"=w378:T18)  [unwired: 1 in, 6 out]
            n233 = call <vilib>:"Close Config Data.vi"("refnum"=w378) -> ("file path"=w379:path)  [unwired: 2 in, 8 out]
            n234 = call <vilib>:"Open Config Data.vi"("configuration file path"=w379) -> ("refnum"=w377:T18)  [unwired: 8 in, 2 out]
          }
          frame True {
            n235 = property on="Camera Settings" class="Clust (strict)"("Visible"=TRUE) -> ()  [unwired: 2 in, 2 out]
          }
        }
      }
      event "Camera Settings": Value Change {
        n236 = event-data() -> ("NewVal"=w408:T1)  [unwired: 1 in]
        n237 = Index Array(array=w404) -> (element=w403:cluster{string[]})  [unwired: 1 in]
        n238 = Unbundle(w408) -> ("Frate Rate"=w399:i32, "Compression"=w398:i32, "Size"=w401:u16)
        n239 = Unbundle(w403) -> (w402:string[])
        n240 = Index Array(array=w402, index=w401) -> (element=w400:string)
        n241 = Format Into String(format string="%s   %dfps   %d%%", w400, w399, w398) -> (resulting string=w405:string)  [unwired: 2 in, 1 out]
        n242 = Build Array(w405) -> (w406:string[])
        n243 = property on="DB Camera Config" class="Bool (strict)"("Strings [4]"=w406) -> ()  [unwired: 2 in, 2 out]
      }
      event "Motor.Enable": Value Change {
        n244 = event-data() -> ("NewVal"=w414:bool)  [unwired: 1 in]
        n245 = Unbundle("Motor") -> ("Value"=w413:dbl)  [unwired: 1 out]
        n246 = Select(t=w413, s=w414, f=0.0) -> (s? t:f=w411:dbl)
        n247 = call <vilib>:"NT Write Number.vi"("Numeric"=w411, "Name"=w410) -> ()  [unwired: 9 in, 1 out]
      }
      event "Slider": Value Change {
        n248 = event-data() -> ("NewVal"=w417:dbl)  [unwired: 1 in]
        n249 = call <vilib>:"NT Write Number.vi"("Numeric"=w417, "Name"=w418) -> ()  [unwired: 9 in, 1 out]
      }
      event "On/Off": Value Change {
        n250 = event-data() -> ("NewVal"=w422:bool)  [unwired: 1 in]
        n251 = Boolean To (0,1)(Boolean=w422) -> (0, 1=w421:i16)
        n252 = call <vilib>:"NT Write Number.vi"("Numeric"=w421, "Name"=w420) -> ()  [unwired: 9 in, 1 out]
      }
      event "Rev/Fwd": Value Change {
        n253 = event-data() -> ("NewVal.Forward"=w430:bool, "NewVal.Reverse"=w429:bool)  [unwired: 1 in]
        n254 = Boolean To (0,1)(Boolean=w430) -> (0, 1=w426:i16)
        n255 = Boolean To (0,1)(Boolean=w429) -> (0, 1=w428:i16)
        n256 = Negate(x=w428) -> (-x=w427:i16)
        n257 = Add(x=w426, y=w427) -> (x+y=w425:i16)
        n258 = call <vilib>:"NT Write Number.vi"("Numeric"=w425, "Name"=w424) -> ()  [unwired: 9 in, 1 out]
      }
      event "Ring": Value Change {
        n259 = event-data() -> ("NewVal"=w434:u16)  [unwired: 1 in]
        n260 = property on="Ring" class="Ring (strict)"() -> ("Strings []"=w435:string[])  [unwired: 2 in, 2 out]
        n261 = Index Array(array=w435, index=w434) -> (element=w433:string)
        n262 = call <vilib>:"NT Write String.vi"("String"=w433, "Name"=w432) -> ()  [unwired: 9 in, 1 out]
      }
    }
  }
  n263 = Index Array(array=w14) -> (element=w15:cluster{string[]})  [unwired: 1 in]
  n264 = Unbundle(w15) -> (w13:string[])
  n265 = Match First String(2:w13, 3:w12) -> (0:w11:i32)  [unwired: 1 out]
  n266 = Bundle("value"=w17, "value"=w16, "index"=w11) -> (w5:cluster{"value":i32, "value":i32, "index":i32})  [unwired: 1 out]
  n267 = property on="On/Off" class="Bool (strict)"("Visible"=w28) -> ()  [unwired: 2 in, 2 out]
  n268 = property on="Motor" class="Clust (strict)"("Visible"=w28) -> ()  [unwired: 2 in, 2 out]
  n269 = property on="Progress" class="Clust (strict)"("Visible"=w28) -> ()  [unwired: 2 in, 2 out]
  n270 = property on="Ring" class="Ring (strict)"("Visible"=w28) -> ()  [unwired: 2 in, 2 out]
  n271 = property on="Camera Settings" class="Clust (strict)"("Val(Sgnl)"=w5) -> ()  [unwired: 2 in, 2 out]
  n272 = property on="Rev/Fwd" class="Clust (strict)"("Visible"=w28) -> ()  [unwired: 2 in, 2 out]
  n273 = property on="Camera Settings" class="Clust (strict)"("Visible"=w28) -> ()  [unwired: 2 in, 2 out]
  n274 = local write "DB Camera Config"(w28) -> ()
